vi "Set Server State UE.vi"(10 "Server State UE":refnum<user-event>, 11 "Template Server in":refnum<class "NW and PSD_server.lvclass">) -> (3 "Template Server out":refnum<class "NW and PSD_server.lvclass">)   [LabVIEW 2019, in "NW and PSD_server.lvlib" / "NW and PSD_server.lvclass"]
uses:
  NW and PSD_server.lvclass
  typeDefs/Server State Data.ctl
  NW and PSD_server.lvclass/NW and PSD_server.ctl
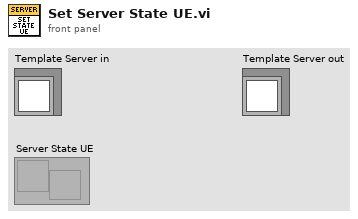
[diagram p1: front panel]
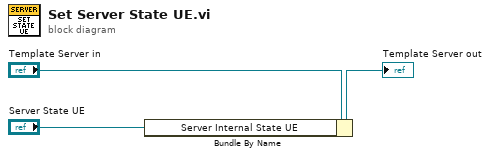
[diagram p0: block diagram]
diagram:
  n1 = Bundle By Name(cluster="Template Server in", "Server Internal State UE"="Server State UE") -> (→"Template Server out":refnum<class "NW and PSD_server.lvclass">)
